vi "Arduino Analog Read Pin Benchmark.vi"() -> ()   [LabVIEW 2011]
doc: "An example that reads a user selectable analog input pin on the Arduino."
uses:
  <vilib>/LabVIEW Interface for Arduino/Private/Type Defs/Analog Pin.ctl
  <vilib>/LabVIEW Interface for Arduino/LabVIEW Interface for Arduino.lvlib
panel:
  out "Update Frequency":dbl
  in  "Analog Pin":T1
  in  "Stop":bool
  out "Voltage":dbl(knob) scale=0.0..5.0
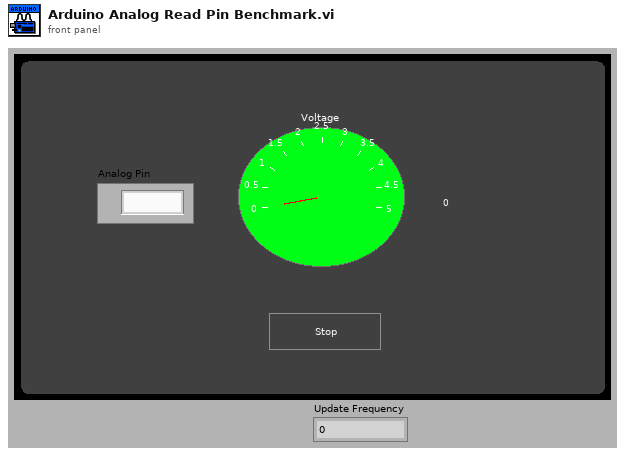
[diagram p1: front panel]
types:
  T1 = typedef "LabVIEW Interface for Arduino.lvlib/Analog Pin.ctl" = enum8{"AI_0", "AI_1", "AI_2", "AI_3", "AI_4", "AI_5", "AI_6", "AI_7", "AI_8", "AI_9", "AI_10", "AI_11", "AI_12", "AI_13", "AI_14", "AI_15"}
  T2 = typedef "LabVIEW Interface for Arduino.lvlib/Arduino Resource.ctl" = cluster{"VISA resource":refnum<visa-resource-name>, "Board Type":T3, "Connection Type":enum8{"USB / Serial"}, "Bytes Per Packet (15)":u8}
  T3 = typedef "LabVIEW Interface for Arduino.lvlib/Board Type.ctl" = enum16{"Arduino Uno", "Dimuelanove w/Atmega 328", "Mega 2560", "Chipkit Uno32", "Chipkit Max32"}
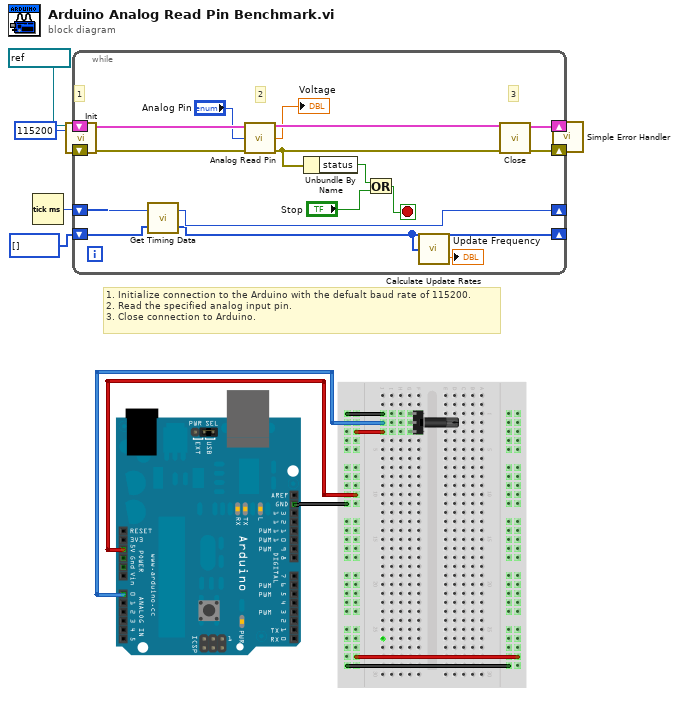
[diagram p0: block diagram]
diagram:
  # "1. Initialize connection to the Arduino with the defualt baud rate of 115200.\n2. Read the specified analog input pin.\n3. Close connection to Arduino."
  # "3"
  # "1"
  n1 = Tick Count (ms)() -> (millisecond timer value=w2:u32)
  n2 = call <vilib>:"Init.vi"("VISA resource"=refnum<visa-resource-name> "COM8", "Baud Rate (115200)"=u32 115200) -> ("Arduino Resource"=w9:T2, "error out"=w6:errorcluster)  [unwired: 16 in]
  n3 = while {
    shift-right: [w23] -> w8
    shift-left: w9 -> [w17]
    shift-right: [w21] -> w7
    shift-left: w6 -> [w16]
    shift-right: [w13] -> _
    shift-left: w2 -> [w14]
    shift-right: [w11] -> _
    shift-left: i32[] [] ("Previous Timing Data") -> [w12]
    stop <- w20 stop-if-true
    # "2"
    n4 = call <vilib>:"Get Timing Data.vi"("Previous Timing Data"=w12, "Previous Tick Count"=w14) -> ("Timing Data"=w11:i32[], "Tick Count"=w13:u32)
    n5 = call <vilib>:"Analog Read Pin.vi"("Arduino Resource"=w17, "Analog Pin"="Analog Pin", "error in"=w16) -> ("Arduino Resource"=w23:T2, "Voltage"=→"Voltage":dbl, "error out"=w21:errorcluster)  [unwired: 10 in]
    n6 = Unbundle By Name(w21) -> ("status"=w19:bool)
    n7 = Or(x=w19, y="Stop") -> (x .or. y?=w20:bool)
    n8 = call <vilib>:"Calculate Update Rates.vi"("Timing Data"=w11) -> ("Update Frequency"=→"Update Frequency":dbl)  [unwired: 1 out]
  }
  n9 = call <vilib>:"Close.vi"("Arduino Resource"=w8, "error in"=w7) -> ("error out"=w5:errorcluster)  [unwired: 13 in]
  n10 = call <vilib>:"Simple Error Handler.vi"("error in (no error)"=w5) -> ()  [unwired: 4 in, 5 out]
